vi "Initialize Variables.vi"(8 "error in":errorcluster) -> (0 "error out":errorcluster)   [LabVIEW 2011]
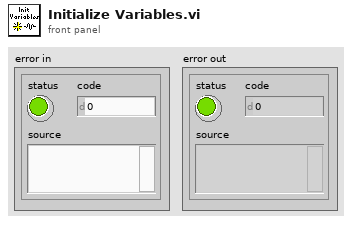
[diagram p1: front panel]
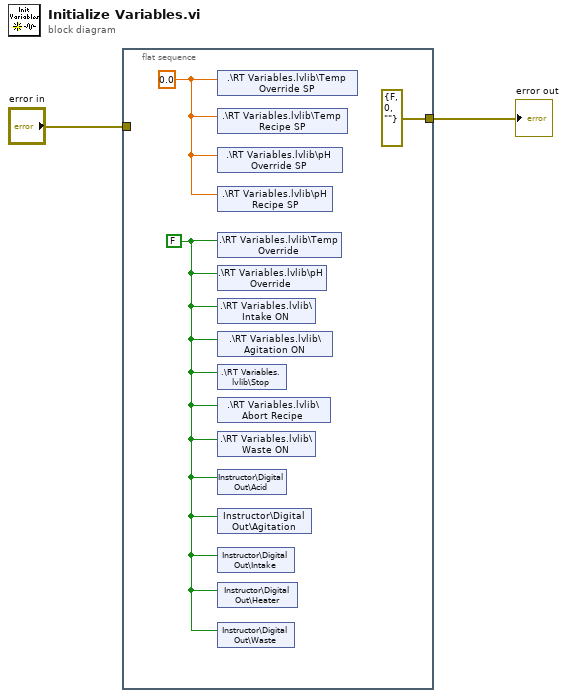
[diagram p0: block diagram]
diagram:
  n1 = flat-sequence {
    tunnel: [errorcluster {"status"=FALSE, "code"=0, "source"=""} ("error in (no error)")] -> w1
    tunnel: "error in" -> [_]
    frame #0 {
      w3 = FALSE
      w4 = 0.0 ("Temp Recipe SP")
      n2 = shared-variable ".\\RT Variables.lvlib\\Temp Override SP"(w4) -> ()  [unwired: 1 in, 1 out]
      n3 = shared-variable ".\\RT Variables.lvlib\\Temp Recipe SP"(w4) -> ()  [unwired: 1 in, 1 out]
      n4 = shared-variable ".\\RT Variables.lvlib\\pH Override SP"(w4) -> ()  [unwired: 1 in, 1 out]
      n5 = shared-variable ".\\RT Variables.lvlib\\pH Recipe SP"(w4) -> ()  [unwired: 1 in, 1 out]
      n6 = shared-variable ".\\RT Variables.lvlib\\Temp Override"(w3) -> ()  [unwired: 1 in, 1 out]
      n7 = shared-variable ".\\RT Variables.lvlib\\pH Override"(w3) -> ()  [unwired: 1 in, 1 out]
      n8 = shared-variable ".\\RT Variables.lvlib\\Intake ON"(w3) -> ()  [unwired: 1 in, 1 out]
      n9 = shared-variable ".\\RT Variables.lvlib\\Agitation ON"(w3) -> ()  [unwired: 1 in, 1 out]
      n10 = shared-variable ".\\RT Variables.lvlib\\Stop"(w3) -> ()  [unwired: 1 in, 1 out]
      n11 = shared-variable ".\\RT Variables.lvlib\\Abort Recipe"(w3) -> ()  [unwired: 1 in, 1 out]
      n12 = shared-variable ".\\RT Variables.lvlib\\Waste ON"(w3) -> ()  [unwired: 1 in, 1 out]
      n13 = shared-variable "Instructor\\Digital Out\\Acid"(w3) -> ()  [unwired: 1 in, 1 out]
      n14 = shared-variable "Instructor\\Digital Out\\Agitation"(w3) -> ()  [unwired: 1 in, 1 out]
      n15 = shared-variable "Instructor\\Digital Out\\Intake"(w3) -> ()  [unwired: 1 in, 1 out]
      n16 = shared-variable "Instructor\\Digital Out\\Heater"(w3) -> ()  [unwired: 1 in, 1 out]
      n17 = shared-variable "Instructor\\Digital Out\\Waste"(w3) -> ()  [unwired: 1 in, 1 out]
    }
  }
  "error out" <- w1
